vi "19052_pass_fail_parser.vi"(8 "error in (no error)":errorcluster, 11 "VISA resource in":refnum<visa-resource-name>) -> (0 "error out":errorcluster, 1 "Pass/Fail":cluster{"PASS":bool, "FAIL":bool}, 2 "Code Results":string, 3 "VISA resource out":refnum<visa-resource-name>)   [LabVIEW 2015]
panel:
  # "This is valid for both:\n19572 & 19052"
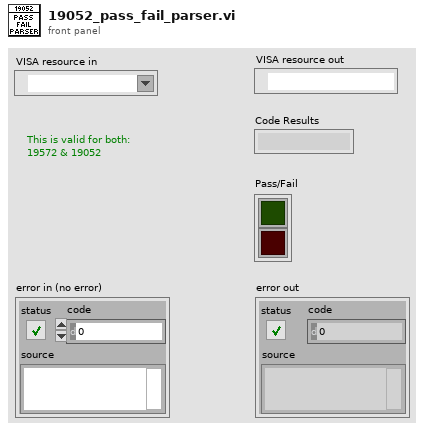
[diagram p1: front panel]
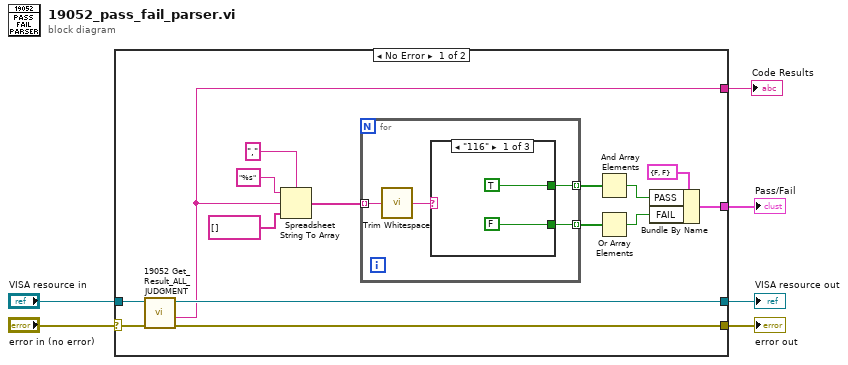
[diagram p0: block diagram]
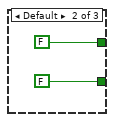
[diagram p2: hidden frame]
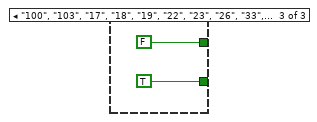
[diagram p3: hidden frame]
diagram:
  n1 = case shown="No Error" "error in (no error)" {
    selector: "error in (no error)" -> [w15 w32]
    tunnel: "VISA resource in" -> [w21 w33]
    tunnel: [w17 w33] -> w5
    tunnel: [w16 w32] -> w4
    tunnel: [w8 _] -> w2
    tunnel: [w7 _] -> w1
    frame No Error {
      n2 = call "19052 Get_Result_ALL_JUDGMENT.vi"("error in (no error)"=w15, "VISA resource in"=w21) -> ("error out"=w16:errorcluster, "JUDGMENT"=w7:string, "VISA resource out"=w17:refnum<visa-resource-name>)  [unwired: 7 in]
      n3 = Spreadsheet String To Array(delimiter (Tab)=",", format string="%s", spreadsheet string=w7, array type (2D Dbl)=string[] []) -> (array=w14:string[])
      n4 = for {
        tunnel: w14 -> [w25] mode=indexing
        tunnel: [w24] -> w13 mode=indexing
        tunnel: [w23] -> w12 mode=indexing
        n5 = call <vilib>:"Trim Whitespace.vi"("string"=w25) -> ("trimmed string"=w22:string)  [unwired: 1 in]
        n6 = case shown="\"116\"" w22 {
          tunnel: [FALSE FALSE TRUE] -> w24
          tunnel: [TRUE FALSE FALSE] -> w23
          frame "116" {
          }
          frame Default {
          }
          frame "100", "103", "17", "18", "19", "22", "23", "26", "33", "34", "35", "37", "38", "39", "49", "50", "54", "55", "97", "98" {
          }
        }
      }
      n7 = And Array Elements(Boolean array=w12) -> (logical AND=w10:bool)
      n8 = Or Array Elements(Boolean array=w13) -> (logical OR=w9:bool)
      n9 = Bundle By Name(cluster=cluster{"PASS":bool, "FAIL":bool} {"PASS"=FALSE, "FAIL"=FALSE} ("Result"), "PASS"=w10, "FAIL"=w9) -> (w8:cluster{"PASS":bool, "FAIL":bool})
    }
    frame Error {
    }
  }
  "VISA resource out" <- w5
  "error out" <- w4
  "Pass/Fail" <- w2
  "Code Results" <- w1
